vi "TDMS Display Defragmentation Progress.vi"() -> ()   [LabVIEW 2023]
doc: "This example demonstrates how to defragment a .tdms file and to display the defragmentation progress."
panel:
  out "Defragmentation Progress (%)":dbl(slide) scale=0.0..100.0
  # "Overview: Demonstrates the progress of defragmenting a .tdms file.\nInstructions:\n1. Run this VI. Note: The defragmentation process may take several seconds to begin displaying its progress.\n2. Delete the .tdms file (located at [LabVIEW Data]\\Example Defragment with Progress Displayed.tdms) when you are done."
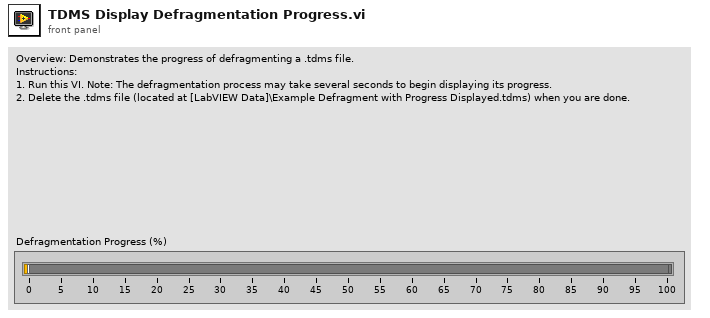
[diagram p1: front panel]
types:
  T1 = enum16{"open", "open or create", "create or replace", "create", "open (read-only)"}
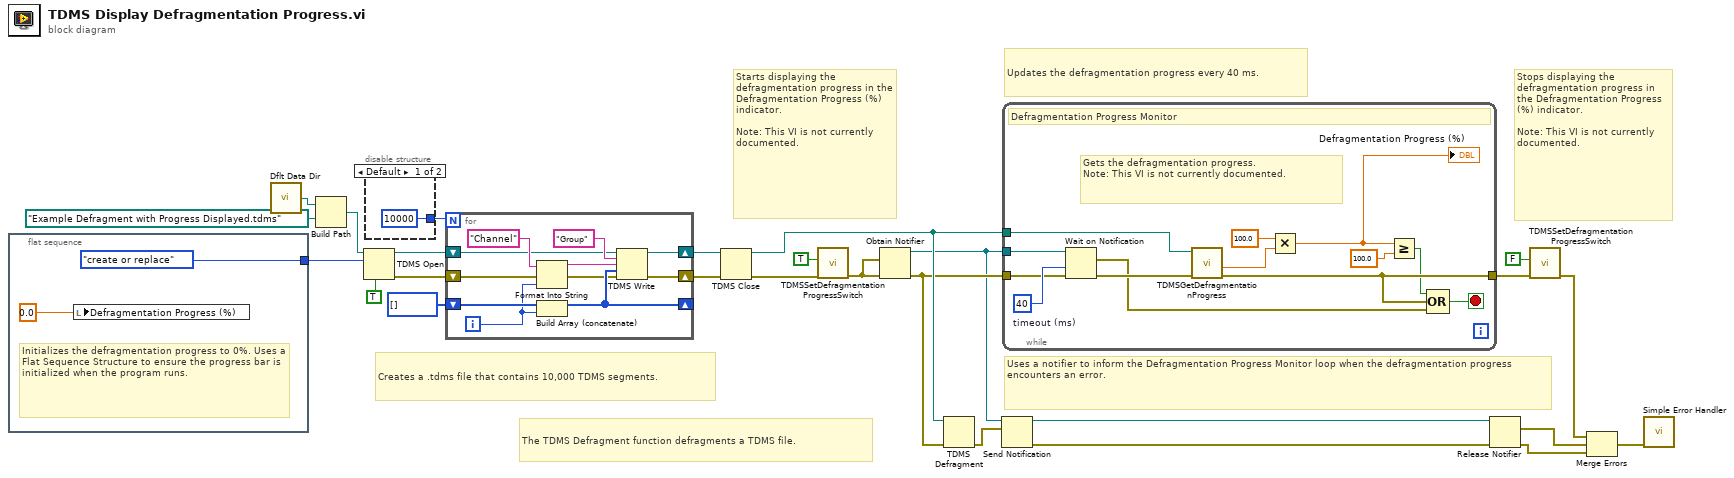
[diagram p0: block diagram]
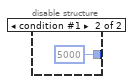
[diagram p2: hidden frame]
diagram:
  # "Uses a notifier to inform the Defragmentation Progress Monitor loop when the defragmentation progress encounters an error."
  # "The TDMS Defragment function defragments a TDMS file."
  # "Stops displaying the defragmentation progress in the Defragmentation Progress (%) indicator.\n\nNote: This VI is not currently documented."
  # "Updates the defragmentation progress every 40 ms."
  # "Starts displaying the defragmentation progress in the Defragmentation Progress (%) indicator.\n\nNote: This VI is not currently documented."
  # "Creates a .tdms file that contains 10,000 TDMS segments."
  n1 = flat-sequence {
    tunnel: [T1."create or replace" ("operation")] -> w25
    frame #0 {
      # "Initializes the defragmentation progress to 0%. Uses a Flat Sequence Structure to ensure the progress bar is initialized when the program runs."
      n2 = local write "Defragmentation Progress (%)"(0.0 ("completionRate")) -> ()
    }
  }
  n3 = call <vilib>:"Dflt Data Dir.vi"() -> ("App:Default Data Directory"=w17:path)
  n4 = Build Path(base path=w17, name or relative path=path "Example Defragment with Progress Displayed.tdms" ("file path")) -> (appended path=w13:path)
  n5 = TDMS Open(6:TRUE ("disable buffering (T)"), 10:w25, 11:w13) -> (0:w18:errorcluster, 3:w20:refnum<k34>)  [unwired: 4 in]
  n6 = disable-structure shown="Default" {
    disable-tunnel: [10000 5000] -> w22
    frame condition #0 (active) {
    }
    frame condition #1 {
    }
  }
  n7 = for {
    N: w22 -> [_]
    shift-right: [w38] -> _
    shift-left: i32[] [] -> [w39]
    shift-right: [w31] -> w14
    shift-left: w18 -> [w33]
    shift-right: [w35] -> w19
    shift-left: w20 -> [w36]
    i -> [w32]
    n8 = Format Into String(initial string="Channel", error in=w33, w32) -> (resulting string=w37:string, error out=w34:errorcluster)  [unwired: 1 in]
    n9 = Build Array (concatenate)(w39, w32) -> (w38:i32[])
    n10 = TDMS Write(0:w36, 5:"Group" ("group name in (Untitled)"), 7:w37, 9:w38, 11:w34) -> (4:w35:refnum<k34>, 15:w31:errorcluster)  [unwired: 1 in, 2 out]
  }
  n11 = TDMS Close(8:w14, 11:w19) -> (0:w16:errorcluster, 3:w26:path)
  n12 = call <vilib>:"TDMSSetDefragmentationProgressSwitch.vi"("error in (no error)"=w16, "display defragmentation progress"=TRUE ("displaySwitch")) -> ("error out"=w4:errorcluster)  [unwired: 7 in]
  n13 = Obtain Notifier(notification data type=w4, error in (no error)=w4) -> (notifier out=w8:refnum<notifier>, error out=w9:errorcluster)  [unwired: 2 in, 1 out]
  n14 = TDMS Defragment(4:w9, 7:w26) -> (0:w3:errorcluster)
  n15 = Send Notification(notification=w3, notifier=w8) -> (notifier out=w6:refnum<notifier>, error out=w7:errorcluster)  [unwired: 1 in]
  n16 = while "Defragmentation Progress Monitor" {
    tunnel: [w48] -> w12
    tunnel: w26 -> [w54]
    tunnel: w9 -> [w50]
    tunnel: w8 -> [w52]
    stop <- w53 stop-if-true
    w51 = 40  # timeout (ms)
    # "Gets the defragmentation progress.\nNote: This VI is not currently documented."
    # "Defragmentation Progress Monitor"
    n17 = Wait on Notification(notifier=w52, timeout in ms (-1)=w51, error in (no error)=w50) -> (notification=w47:errorcluster, error out=w49:errorcluster)  [unwired: 1 in, 2 out]
    n18 = call <vilib>:"TDMSGetDefragmentationProgress.vi"("error in (no error)"=w49, "file path in"=w54) -> ("error out"=w48:errorcluster, "progress"=w45:dbl)  [unwired: 5 in, 1 out]
    n19 = Multiply(x=100.0, y=w45) -> (x*y=w44:dbl)
    "Defragmentation Progress (%)" <- w44
    n20 = Greater Or Equal?(x=w44, y=100.0) -> (x >= y?=w42:bool)
    n21 = Compound Arithmetic op=OR(w42, w48, w47) -> (w53:bool)
  }
  n22 = Release Notifier(notifier=w6, error in (no error)=w7) -> (last notification=w2:errorcluster, error out=w1:errorcluster)  [unwired: 1 in, 1 out]
  n23 = call <vilib>:"TDMSSetDefragmentationProgressSwitch.vi"("error in (no error)"=w12, "display defragmentation progress"=FALSE ("displaySwitch")) -> ("error out"=w11:errorcluster)  [unwired: 7 in]
  n24 = Merge Errors(w11, w2, w1) -> (w5:errorcluster)
  n25 = call <vilib>:"Simple Error Handler.vi"("error in (no error)"=w5) -> ()  [unwired: 2 in, 7 out]
